vi "Build Config File From Part Config.vi"(7 "Loaded Config":T1={"DAQ Settings"={"Trigger Type"=enum."Manual", "Trigger Samples"=0, "Pretrigger Samples"=0, "Trigger Interval"=0.0, "Time Units"=FALSE, "Auto Save"=FALSE, "Sample Rate"=7.0, "Select Analog"=FALSE, "Trigger Value"=0.0, "Trigger Stop Method"=enum."Use Samples Value to Stop Trigger", "Rate Sec/Min"=FALSE, "Save Mode"=enum."Single File", "File Size Limit"=0.0, "Log File Type"=enum."Basic", "Trigger Data Index"=0}, "Channels"=[], "Header"={"TA Number"="", "Test Name"="", "Serial Number"="", "Technician"=""}, "Graph Settings"={"Graph Labels"=[], [], [], [], [], [], [], [], [], [], [], [], [], "Graph Toggles"=[], "Axis Toggles"=[], "Graph Range"=enum."1"}, "Test Limits"=[], "All Type Info"=[], "Save Mode"=enum."Single File"} {"DAQ Settings"."Trigger Interval" min=0.0; "DAQ Settings"."Pretrigger Samples" min=0; "DAQ Settings"."Trigger Samples" min=0}, 9 "All Test Limits":cluster{T8[]}[](array[cluster]), 10 "All Type Info":T9, 11 "Config In":T1={"DAQ Settings"={"Trigger Type"=enum."Manual", "Trigger Samples"=0, "Pretrigger Samples"=0, "Trigger Interval"=0.0, "Time Units"=FALSE, "Auto Save"=FALSE, "Sample Rate"=7.0, "Select Analog"=FALSE, "Trigger Value"=0.0, "Trigger Stop Method"=enum."Use Samples Value to Stop Trigger", "Rate Sec/Min"=FALSE, "Save Mode"=enum."Single File", "File Size Limit"=0.0, "Log File Type"=enum."Basic", "Trigger Data Index"=0}, "Channels"=[], "Header"={"TA Number"="", "Test Name"="", "Serial Number"="", "Technician"=""}, "Graph Settings"={"Graph Labels"=[], [], [], [], [], [], [], [], [], [], [], [], [], "Graph Toggles"=[], "Axis Toggles"=[], "Graph Range"=enum."1"}, "Test Limits"=[], "All Type Info"=[], "Save Mode"=enum."Single File"} {"DAQ Settings"."Trigger Interval" min=0.0; "DAQ Settings"."Pretrigger Samples" min=0; "DAQ Settings"."Trigger Samples" min=0}) -> (3 "Config Out":T1={"DAQ Settings"={"Trigger Type"=enum."Manual", "Trigger Samples"=0, "Pretrigger Samples"=0, "Trigger Interval"=0.0, "Time Units"=FALSE, "Auto Save"=FALSE, "Sample Rate"=7.0, "Select Analog"=FALSE, "Trigger Value"=0.0, "Trigger Stop Method"=enum."Use Samples Value to Stop Trigger", "Rate Sec/Min"=FALSE, "Save Mode"=enum."Single File", "File Size Limit"=0.0, "Log File Type"=enum."Basic", "Trigger Data Index"=0}, "Channels"=[], "Header"={"TA Number"="", "Test Name"="", "Serial Number"="", "Technician"=""}, "Graph Settings"={"Graph Labels"=[], [], [], [], [], [], [], [], [], [], [], [], [], "Graph Toggles"=[], "Axis Toggles"=[], "Graph Range"=enum."1"}, "Test Limits"=[], "All Type Info"=[], "Save Mode"=enum."Single File"} {"DAQ Settings"."Trigger Interval" min=0.0; "DAQ Settings"."Pretrigger Samples" min=0; "DAQ Settings"."Trigger Samples" min=0})   [LabVIEW 2019]
uses:
  Type Defs and Controls/Test Limits.ctl
  Type Defs and Controls/All Part Info.ctl
  Type Defs and Controls/Part Info.ctl
  Type Defs and Controls/Sensor Config.ctl
  Type Defs and Controls/DAQ Settings.ctl
  Type Defs and Controls/Trigger Stop Method.ctl
  Type Defs and Controls/Log File Type.ctl
  Type Defs and Controls/Channel Config.ctl
  Type Defs and Controls/Header.ctl
  Type Defs and Controls/Graph Settings Type Def.ctl
panel:
  # "EGU"
  # "EGU"
  # "EGU"
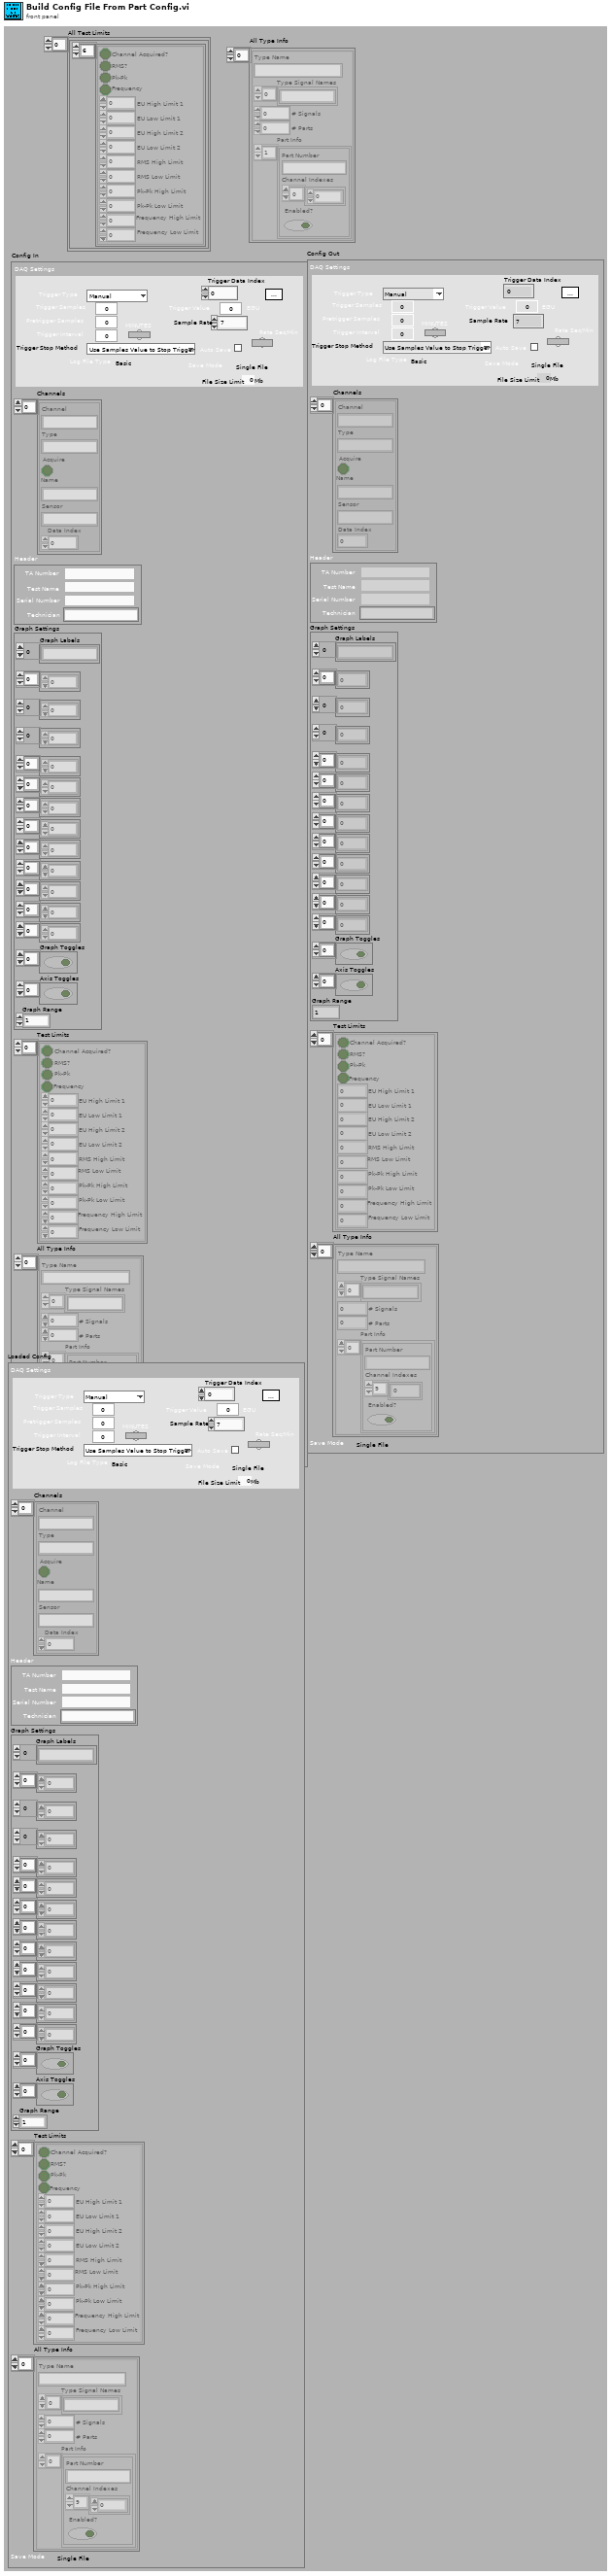
[diagram p1: front panel]
types:
  T1 = typedef "Sensor Config.ctl" = cluster{"DAQ Settings":T2, "Channels":T5[], "Header":T6, "Graph Settings":T7, "Test Limits":T8[], "All Type Info":T9, "Save Mode":enum16{"Single File", "Segmented Files", "New File at Midnight"}}
  T2 = typedef "DAQ Settings.ctl" = cluster{"Trigger Type":enum16{"Manual", "Timed", "Analog Rising", "Analog Falling"}, "Trigger Samples":i32, "Pretrigger Samples":i32, "Trigger Interval":dbl, "Time Units":bool, "Auto Save":bool, "Sample Rate":dbl, "Select Analog":bool, "Trigger Value":dbl, "Trigger Stop Method":T3, "Rate Sec/Min":bool, "Save Mode":enum16{"Single File", "Segmented Files", "New File at Midnight"}, "File Size Limit":dbl, "Log File Type":T4, "Trigger Data Index":u32}
  T3 = typedef "Trigger Stop Method.ctl" = enum16{"Use Samples Value to Stop Trigger", "Use Threshold to Stop Trigger"}
  T4 = typedef "Log File Type.ctl" = enum16{"Basic", "RTS"}
  T5 = typedef "Channel Config.ctl" = cluster{"Channel":string, "Type":string, "Acquire":bool, "Name":string, "Sensor":string, "Data Index":u32}
  T6 = typedef "Header.ctl" = cluster{"TA Number":string, "Test Name":string, "Serial Number":string, "Technician":string}
  T7 = typedef "Graph Settings Type Def.ctl" = cluster{"Graph Labels":string[], u8[], i16[], u32[], u8[], u8[], u8[], u32[], u8[], u8[], u8[], dbl[], dbl[], "Graph Toggles":bool[], "Axis Toggles":bool[], "Graph Range":enum16{"1", "2", "3", "4", "5", "10", "15", "30", "60"}}
  T8 = typedef "Test Limits.ctl" = cluster{"Channel Acquired?":bool, "RMS?":bool, "Pk-Pk":bool, "Frequency":bool, "EU High Limit 1":dbl, "EU Low Limit 1":dbl, "EU High Limit 2":dbl, "EU Low Limit 2":dbl, "RMS High Limit":dbl, "RMS Low Limit":dbl, "Pk-Pk High Limit ":dbl, "Pk-Pk Low Limit":dbl, "Frequency High Limit":dbl, "Frequency Low Limit":dbl}
  T9 = typedef "All Part Info.ctl" = cluster{"Type Name":string, "Type Signal Names":string[], "# Signals":i32, "# Parts":i32, "Part Info":T10[]}[]
  T10 = typedef "Part Info.ctl" = cluster{"Part Number":string, "Channel Indexes":u16[], "Enabled?":bool}
  T11 = cluster{"Type Name":string, "Type Signal Names":string[], "# Signals":i32, "# Parts":i32, "Part Info":T10[]}
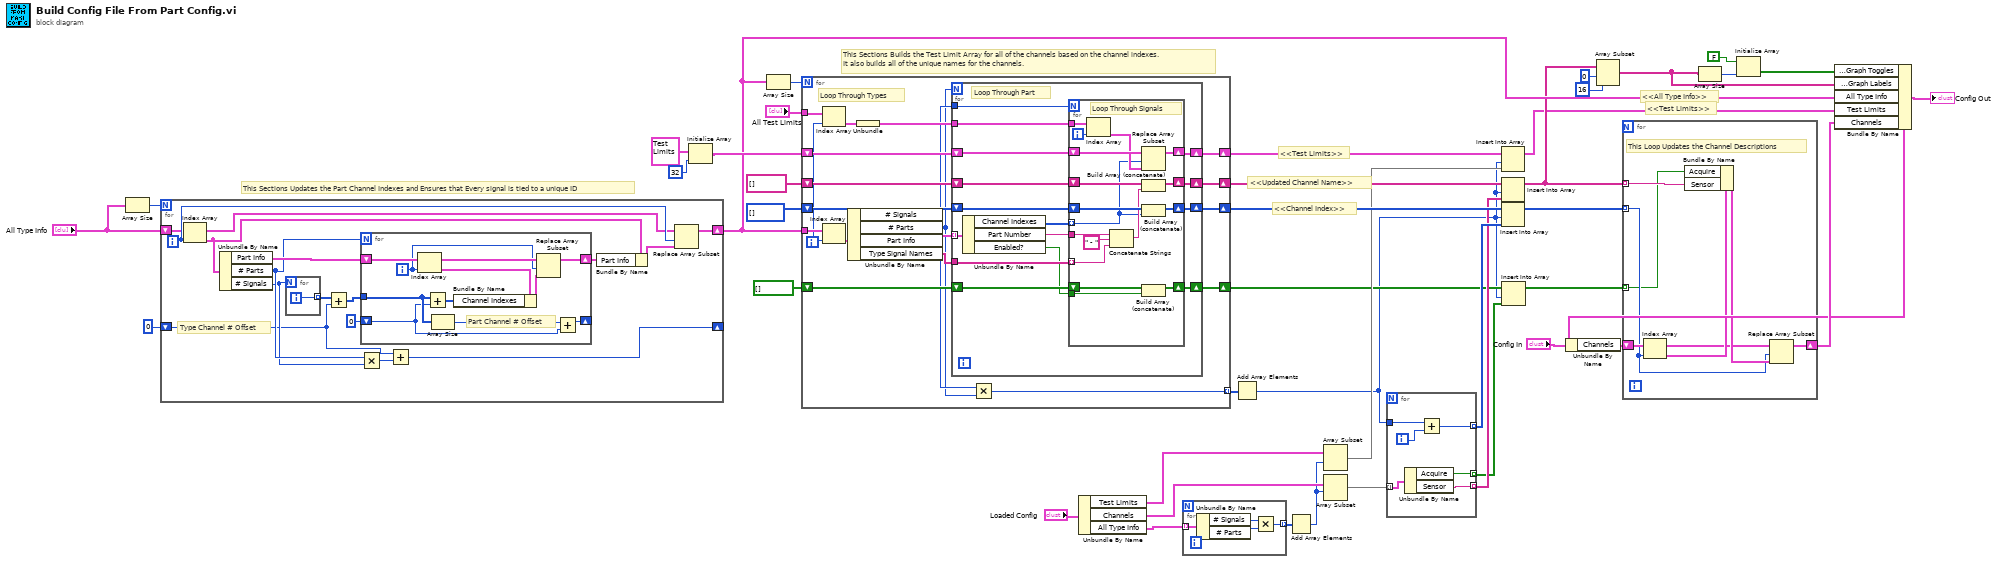
[diagram p0: block diagram]
diagram:
  # "<<All Type Info>>"
  # "<<Test Limits>>"
  # "<<Test Limits>>"
  # "<<Channel Index>>"
  # "<<Updated Channel Name>>"
  # "This Sections Builds the Test Limit Array for all of the channels based on the channel indexes.\nIt also builds all of the unique names for the channels."
  # "This Sections Updates the Part Channel Indexes and Ensures that Every signal is tied to a unique ID"
  n1 = Array Size(array="All Type Info") -> (size(s)=w39:i32)
  n2 = for {
    N: w39 -> [_]
    shift-right: [w57] -> w29
    shift-left: "All Type Info" -> [w55]
    shift-right: [w45] -> _
    shift-left: 0 -> [w44]
    i -> [w56]
    # "Type Channel # Offset"
    n3 = Index Array(array=w55, index=w56) -> (element=w54:T11)
    n4 = Unbundle By Name(w54) -> ("Part Info"=w58:T10[], "# Parts"=w48:i32, "# Signals"=w47:i32)
    n5 = for {
      N: w47 -> [_]
      tunnel: [w69] -> w51 mode=indexing
      i -> [w69]
    }
    n6 = Add(x=w51, y=w44) -> (x+y=w49:i32[])
    n7 = Multiply(x=w48, y=w47) -> (x*y=w46:i32)
    n8 = for {
      N: w48 -> [_]
      tunnel: w49 -> [w62]
      shift-right: [w60] -> _
      shift-left: 0 -> [w59]
      shift-right: [w64] -> w52
      shift-left: w58 -> [w65]
      i -> [w63]
      # "Part Channel # Offset"
      n9 = Index Array(array=w65, index=w63) -> (element=w67:T10)
      n10 = Add(x=w62, y=w59) -> (x+y=w68:i32[])
      n11 = Array Size(array=w62) -> (size(s)=w61:i32)
      n12 = Bundle By Name(cluster=w67, "Channel Indexes"=w68) -> (w66:T10)
      n13 = Replace Array Subset(array=w65, new element=w66, index=w63) -> (w64:T10[])
      n14 = Add(x=w61, y=w59) -> (x+y=w60:i32)
    }
    n15 = Add(x=w44, y=w46) -> (x+y=w45:i32)
    n16 = Bundle By Name(cluster=w54, "Part Info"=w52) -> (w53:T11)
    n17 = Replace Array Subset(array=w55, new element=w53, index=w56) -> (w57:T9)
  }
  n18 = Initialize Array(T8 {"Channel Acquired?"=FALSE, "RMS?"=FALSE, "Pk-Pk"=FALSE, "Frequency"=FALSE, "EU High Limit 1"=0.0, "EU Low Limit 1"=0.0, "EU High Limit 2"=0.0, "EU Low Limit 2"=0.0, "RMS High Limit"=0.0, "RMS Low Limit"=0.0, "Pk-Pk High Limit "=0.0, "Pk-Pk Low Limit"=0.0, "Frequency High Limit"=0.0, "Frequency Low Limit"=0.0} ("Test Limit"), 32 ("dimension size")) -> (w35:T8[])
  n19 = Array Size(array=w29) -> (size(s)=w41:i32)
  n20 = for {
    N: w41 -> [_]
    tunnel: w29 -> [w88]
    shift-right: [w82] -> w27
    shift-left: string[] [] -> [w83]
    shift-right: [w81] -> w34
    shift-left: u16[] [] ("Channel Indexes") -> [w84]
    shift-right: [w75] -> w10
    shift-left: w35 -> [w80]
    tunnel: "All Test Limits" -> [w79]
    shift-right: [w73] -> w6
    shift-left: bool[] [] -> [w74]
    tunnel: [w70] -> w16 mode=indexing
    i -> [w78]
    # "Loop Through Types"
    n21 = Index Array(array=w79, index=w78) -> (element=w77:cluster{T8[]})
    n22 = Index Array(array=w88, index=w78) -> (element=w87:T11)
    n23 = Unbundle By Name(w87) -> ("# Signals"=w72:i32, "# Parts"=w71:i32, "Part Info"=w86:T10[], "Type Signal Names"=w85:string[])
    n24 = Unbundle(w77) -> (w76:T8[])
    n25 = for {
      N: w71 -> [_]
      tunnel: w86 -> [w102] mode=indexing
      tunnel: w85 -> [w103]
      shift-right: [w96] -> w81
      shift-left: w84 -> [w99]
      shift-right: [w97] -> w82
      shift-left: w83 -> [w98]
      shift-right: [w93] -> w75
      shift-left: w80 -> [w94]
      tunnel: w76 -> [w95]
      shift-right: [w90] -> w73
      shift-left: w74 -> [w92]
      tunnel: w72 -> [w89]
      # "Loop Through Part"
      n26 = Unbundle By Name(w102) -> ("Channel Indexes"=w101:u16[], "Part Number"=w100:string, "Enabled?"=w91:bool)
      n27 = for {
        N: w89 -> [_]
        tunnel: w103 -> [w118] mode=indexing
        tunnel: w101 -> [w107] mode=indexing
        tunnel: w100 -> [w120]
        shift-right: [w114] -> w97
        shift-left: w98 -> [w116]
        shift-right: [w113] -> w96
        shift-left: w99 -> [w117]
        tunnel: w95 -> [w112]
        shift-right: [w110] -> w93
        shift-left: w94 -> [w111]
        shift-right: [w105] -> w90
        shift-left: w92 -> [w106]
        tunnel: w91 -> [w104]
        i -> [w108]
        # "Loop Through Signals"
        n28 = Index Array(array=w112, index=w108) -> (element=w109:T8)
        n29 = Concatenate Strings(w120, " - " ("string"), w118) -> (w115:string)
        n30 = Replace Array Subset(array=w111, new element=w109, index=w107) -> (w110:T8[])
        n31 = Build Array (concatenate)(w116, w115) -> (w114:string[])
        n32 = Build Array (concatenate)(w117, w107) -> (w113:u16[])
        n33 = Build Array (concatenate)(w106, w104) -> (w105:bool[])
      }
    }
    n34 = Multiply(x=w72, y=w71) -> (x*y=w70:i32)
  }
  n35 = Unbundle By Name("Loaded Config") -> ("Test Limits"=w15:T8[], "Channels"=w18:T5[], "All Type Info"=w20:T9)
  n36 = for {
    tunnel: w20 -> [w124] mode=indexing
    tunnel: [w121] -> w19 mode=indexing
    n37 = Unbundle By Name(w124) -> ("# Signals"=w123:i32, "# Parts"=w122:i32)
    n38 = Multiply(x=w123, y=w122) -> (x*y=w121:i32)
  }
  n39 = Add Array Elements(numeric array=w16) -> (sum=w4:i32)
  n40 = Add Array Elements(numeric array=w19) -> (sum=w14:i32)
  n41 = Array Subset(array=w15, index=w14) -> (w9:T8[])  [unwired: 1 in]
  n42 = Array Subset(array=w18, index=w14) -> (w17:T5[])  [unwired: 1 in]
  n43 = for {
    tunnel: w17 -> [w130] mode=indexing
    tunnel: w4 -> [w128]
    tunnel: [w127] -> w12 mode=indexing
    tunnel: [w126] -> w7 mode=indexing
    tunnel: [w125] -> w3 mode=indexing
    i -> [w129]
    n44 = Unbundle By Name(w130) -> ("Acquire"=w125:bool, "Sensor"=w126:string)
    n45 = Add(x=w128, y=w129) -> (x+y=w127:i32)
  }
  n46 = Insert Into Array(array=w10, index=w4, new element=w9) -> (w8:T8[])
  n47 = Insert Into Array(array=w27, index=w4, new element=w7) -> (w11:string[])
  n48 = Insert Into Array(array=w34, index=w4, new element=w12) -> (w13:u16[])
  n49 = Insert Into Array(array=w6, index=w4, new element=w3) -> (w5:bool[])
  n50 = Unbundle By Name("Config In") -> ("Channels"=w28:T5[])
  n51 = Array Subset(array=w11, index=0, length=16) -> (w24:string[])
  n52 = for {
    tunnel: w11 -> [w134] mode=indexing
    tunnel: w13 -> [w132] mode=indexing
    shift-right: [w133] -> w33
    shift-left: w28 -> [w135]
    tunnel: w5 -> [w131] mode=indexing
    # "This Loop Updates the Channel Descriptions"
    n53 = Index Array(array=w135, index=w132) -> (element=w137:T5)
    n54 = Bundle By Name(cluster=w137, "Acquire"=w131, "Sensor"=w134) -> (w136:T5)
    n55 = Replace Array Subset(array=w135, new element=w136, index=w132) -> (w133:T5[])
  }
  n56 = Array Size(array=w24) -> (size(s)=w23:i32)
  n57 = Initialize Array(FALSE, w23) -> (w21:bool[])
  n58 = Bundle By Name(cluster="Config In", "Graph Settings.Graph Toggles"=w21, "Graph Settings.Graph Labels"=w24, "All Type Info"=w29, "Test Limits"=w8, "Channels"=w33) -> (→"Config Out":T1)
